vi "write macro.vi"(8 "Data byte":u8=2 format="%x", 9 "Reg Address":u8=2 format="%x", 10 "Address":u8=2 format="%x", 11 "Input Port in":T1 items=["Port 1", "Port 2", "Port 3", "Port 4"]) -> (1 "Status":string, 2 "Error":bool, 3 "Input Port out":T1 items=["Port 1", "Port 2", "Port 3", "Port 4"])   [LabVIEW 2016]
uses:
  <vilib>/NXT/Block Support/HWPage.SensorType.ctl
  <vilib>/NXT/Block Support/HWPage.SensorMode.ctl
  <vilib>/NXT/Block Support/NXT_InputPort.ctl
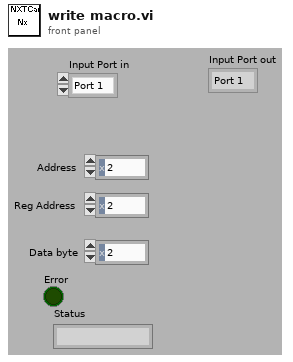
[diagram p1: front panel]
types:
  T1 = typedef "NXT_InputPort.ctl" = u32
  T2 = typedef "HWPage.SensorMode.ctl" = u8
  T3 = typedef "HWPage.SensorType.ctl" = u8
  T4 = typedef "nxt.ctl" = cluster{"nxtHandle":u64, "fileHandle":u64, "fileIterHandle":u64, "moduleHandle":u64, "modIterHandle":u64, "nxtIterHandle":u64}
  T5 = typedef "NXT_StatusCodes.ctl" = i8
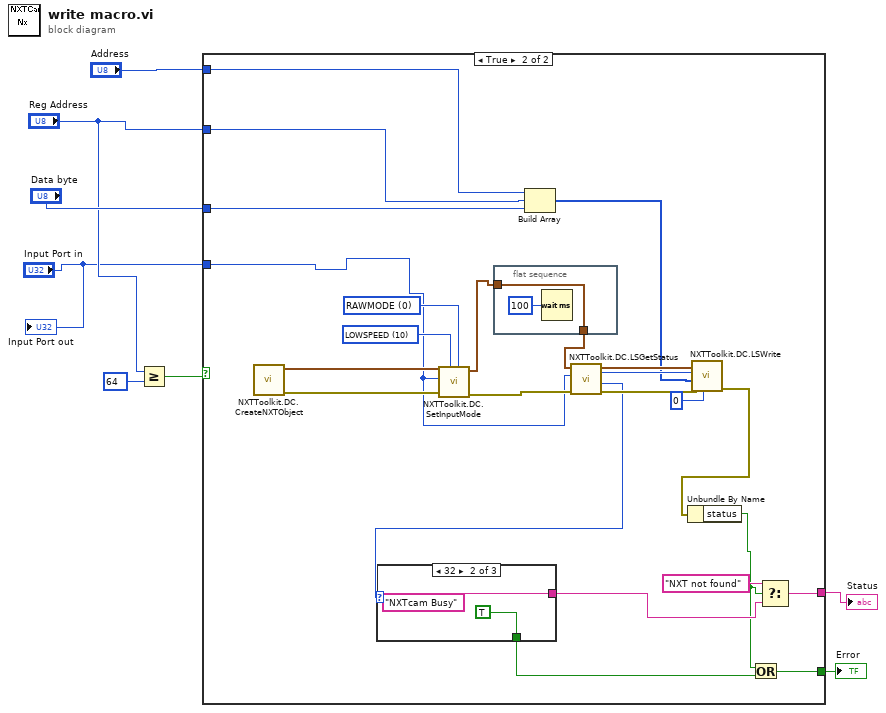
[diagram p0: block diagram]
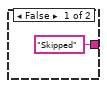
[diagram p2: hidden frame]
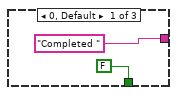
[diagram p3: hidden frame]
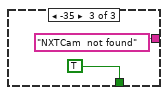
[diagram p4: hidden frame]
diagram:
  n1 = Greater Or Equal?(x="Reg Address", y=u8 64) -> (x >= y?=w2:bool)
  n2 = case shown="True" w2 {
    tunnel: "Address" -> [_ w21]
    tunnel: "Reg Address" -> [_ w20]
    tunnel: "Data byte" -> [_ w19]
    tunnel: ["Skipped" ("t") w12] -> w6
    tunnel: [_ w11] -> w5
    tunnel: "Input Port in" -> [_ w10]
    frame False {
    }
    frame True {
      w32 = T2 0 items=["RAWMODE"=0, "BOOLEANMODE"=32, "TRANSITIONCNTMODE"=64, "PERIODCOUNTERMODE"=96, "PCTFULLSCALEMODE"=128, "CELSIUSMODE"=160, "FAHRENHEITMODE"=192, "ANGLESTEPMODE"=224] ("Sensor Mode (RAWMODE)")
      w33 = T3 10 items=["NO_SENSOR", "SWITCH", "TEMPERATURE", "REFLECTION", "ANGLE", "LIGHT_ACTIVE", "LIGHT_INACTIVE", "SOUND_DB", "SOUND_DBA", "CUSTOM", "LOWSPEED", "LOWSPEED_9V", "HIGHSPEED"] ("Sensor Type (NO_SENSOR)")
      n3 = call <vilib>:"NXTToolkit.DC.CreateNXTObject.vi"() -> ("error out"=w25:errorcluster, "NXTObject"=w26:T4)  [unwired: 9 in, 1 out]
      n4 = call <vilib>:"NXTToolkit.DC.SetInputMode.vi"("Sensor Mode (RAWMODE)"=w32, "Sensor Type (NO_SENSOR)"=w33, "error in (no error)"=w25, "Input Port (Port 1)"=w10, "NXTObject"=w26) -> ("error out"=w31:errorcluster, "NXTObject dup"=w23:T4)  [unwired: 4 in, 1 out]
      n5 = flat-sequence {
        tunnel: [w40] -> w24
        tunnel: w23 -> [w40]
        frame #0 {
          n6 = Wait (ms)(milliseconds to wait=u32 100) -> ()  [unwired: 1 out]
        }
      }
      n7 = Build Array(w21, w20, w19) -> (w22:u8[])
      n8 = call <vilib>:"NXTToolkit.DC.LSGetStatus.vi"("error in (no error)"=w31, "Input Port (Port 1)"=w10, "NXTObject"=w24) -> ("error out"=w29:errorcluster, "Status"=w13:T5, "Input Port dup"=w28:T1, "NXTObject dup"=w30:T4)  [unwired: 2 in, 3 out]
      n9 = case shown="32" w13 {
        tunnel: ["Completed " "NXTcam Busy" "NXTCam  not found"] -> w18
        tunnel: [FALSE TRUE TRUE] -> w16
        frame 0, Default {
        }
        frame 32 {
        }
        frame -35 {
        }
      }
      n10 = call <vilib>:"NXTToolkit.DC.LSWrite.vi"("Response Length (0)"=0, "error in (no error)"=w29, "Buffer"=w22, "Input Port (Port 1)"=w28, "NXTObject"=w30) -> ("error out"=w15:errorcluster)  [unwired: 3 in, 3 out]
      n11 = Unbundle By Name(w15) -> ("status"=w14:bool)
      n12 = Or(x=w14, y=w16) -> (x .or. y?=w11:bool)
      n13 = Select(t="NXT not found", s=w14, f=w18) -> (s? t:f=w12:string)
    }
  }
  "Status" <- w6
  "Error" <- w5
  "Input Port out" <- "Input Port in"
